vi "CLSUIP_GetFPTermPosition.vi"(8 "error in (no error)":errorcluster, 10 "Control Ref":refnum<vi>, 11 "VI Refnum":refnum<vi>) -> (0 "error out":errorcluster, 1 "Position":cluster{"Left":i32, "Top":i32}, 2 "Control Ref out":refnum<vi>, 3 "VI Refnum out":refnum<vi>)   [LabVIEW 2021, in "MemberVICreation.lvlib"]
uses:
  <resource>/Framework/Providers/LVClassLibrary/NewAccessors/MemberVICreation.lvlib
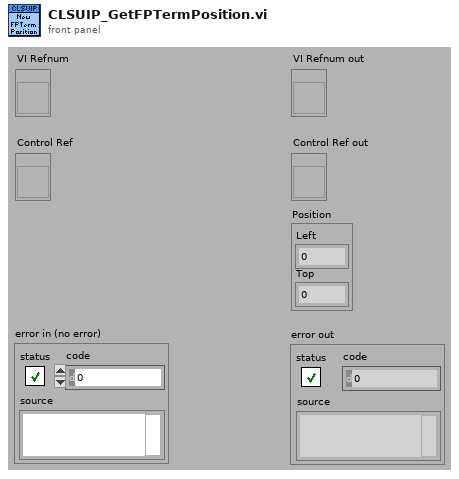
[diagram p1: front panel]
types:
  T1 = typedef "LVRectTypeDef.ctl" = cluster{"left":i16, "top":i16, "right":i16, "bottom":i16}
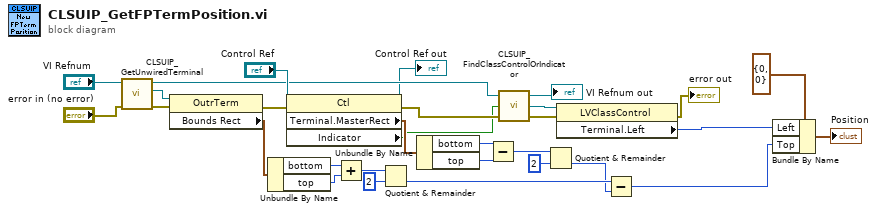
[diagram p0: block diagram]
diagram:
  n1 = call <resource>:"CLSUIP_GetUnwiredTerminal.vi"("error in (no error)"="error in (no error)", "VI Refnum"="VI Refnum") -> ("error out"=w29:errorcluster, "Outer Terminal Ref"=w30:refnum<vi>, "VI Refnum out"=w15:refnum<vi>)  [unwired: 7 out]
  n2 = property class="OutrTerm"(reference=w30, error in=w29) -> (error out=w21:errorcluster, "Bounds Rect"=w28:T1)  [unwired: 1 out]
  n3 = Unbundle By Name(w28) -> ("bottom"=w26:i16, "top"=w27:i16)
  n4 = property class="Ctl"(reference="Control Ref", error in=w21) -> (reference out=→"Control Ref out":refnum<vi>, error out=w16:errorcluster, "Terminal.MasterRect"=w6:T1, "Indicator"=w2:bool)
  n5 = Add(x=w26, y=w27) -> (x+y=w25:i16)
  n6 = Quotient & Remainder(x=w25, y=i16 2) -> (floor(x/y)=w20:i16)  [unwired: 1 out]
  n7 = Unbundle By Name(w6) -> ("bottom"=w4:i16, "top"=w5:i16)
  n8 = Subtract(x=w4, y=w5) -> (x-y=w3:i16)
  n9 = call <resource>:"CLSUIP_FindClassControlOrIndicator.vi"("error in (no error)"=w16, "Indicator?"=w2, "VI Refnum"=w15) -> ("error out"=w13:errorcluster, "LVClassControl Refnum"=w12:refnum<vi>, "VI Refnum out"=→"VI Refnum out":refnum<vi>)
  n10 = Quotient & Remainder(x=w3, y=i16 2) -> (floor(x/y)=w19:i16)  [unwired: 1 out]
  n11 = property class="LVClassControl"(reference=w12, error in=w13) -> (error out=→"error out":errorcluster, "Terminal.Left"=w8:i32)  [unwired: 1 out]
  n12 = Subtract(x=w20, y=w19) -> (x-y=w7:i16)
  n13 = Bundle By Name(cluster=cluster{"Left":i32, "Top":i32} {"Left"=0, "Top"=0} ("Position"), "Left"=w8, "Top"=w7) -> (→"Position":cluster{"Left":i32, "Top":i32})
